vi "configure.vi"(8 "error in (no error)":errorcluster, 9 "Value":i32, 10 "ILC":refnum<class "ILC.lvclass">, 11 "ConfigureILCSSRStrategy in":refnum<class "ConfigureILCDCADAC2Strategy.lvclass">) -> (0 "error out":errorcluster, 2 "ILC 2":refnum<class "ILC.lvclass">, 3 "ConfigureILCSSRStrategy out":refnum<class "ConfigureILCDCADAC2Strategy.lvclass">)   [LabVIEW 2015, in "ConfigureILCDCADAC2Strategy.lvclass"]
uses:
  ConfigureILCDCADAC2Strategy.lvclass
  <userlib>/Common/ILC/ILC/ILC.lvclass
  <userlib>/Common/ILC/ILC/ILC.lvclass/ILC.ctl
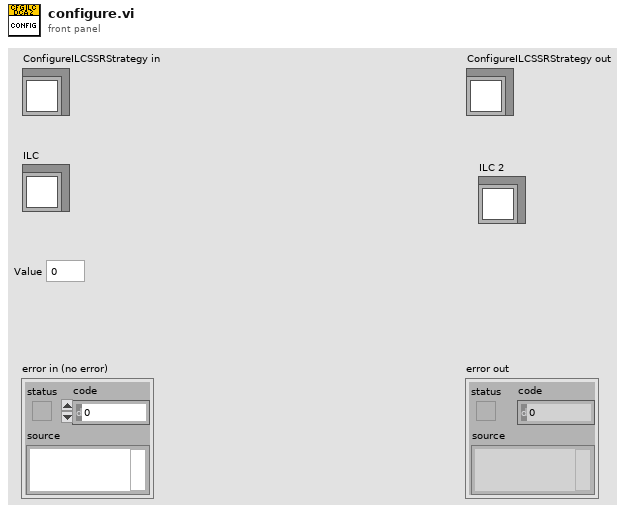
[diagram p1: front panel]
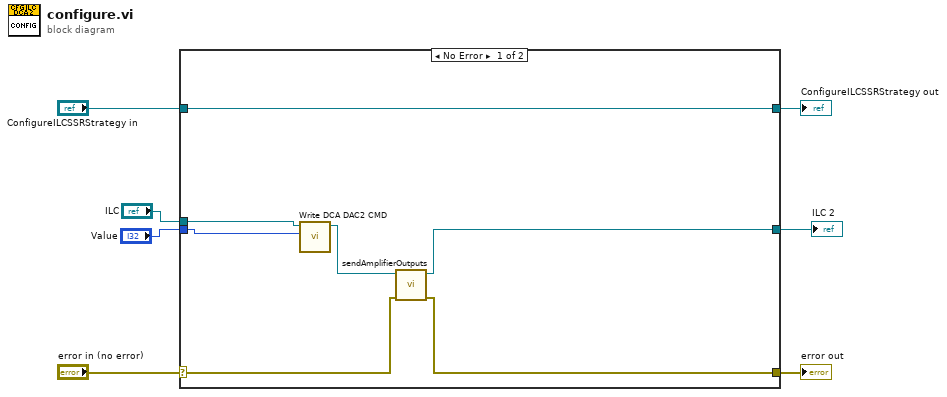
[diagram p0: block diagram]
diagram:
  n1 = case shown="No Error" "error in (no error)" {
    selector: "error in (no error)" -> [w13 w17]
    tunnel: [w12 w17] -> w6
    tunnel: [w14 w16] -> w4
    tunnel: "ConfigureILCSSRStrategy in" -> [w14 w16]
    tunnel: "ILC" -> [w10 w15]
    tunnel: "Value" -> [w9 _]
    tunnel: [w11 w15] -> w1
    frame No Error {
      n2 = call <userlib>:"Write DCA DAC2 CMD.vi"("DCA DAC2 CMD"=w9, "ILC in"=w10) -> ("ILC out"=w8:refnum<class "ILC.lvclass">)  [unwired: 9 in]
      n3 = call <userlib>:"sendAmplifierOutputs.vi"("error in (no error)"=w13, "ILC in"=w8) -> ("error out"=w12:errorcluster, "ILC out"=w11:refnum<class "ILC.lvclass">)  [unwired: 8 in]
    }
    frame Error {
    }
  }
  "error out" <- w6
  "ConfigureILCSSRStrategy out" <- w4
  "ILC 2" <- w1
